vi "Obtain Events.vi"(8 "Error In":errorcluster, 11 "SPD.Stand Ctrl in":T1 {"spdDeviceSession"."hidSPD.Controller"."HV_bias" format="%#_6p, V"; "spdDeviceSession"."hidSPD.Controller"."TSet" format="%#_6p, DegC"}) -> (0 "Error Out":errorcluster, 2 "Event Registration Refnum":refnum<event-registration>, 3 "SPD.Stand Ctrl out":T1 {"spdDeviceSession"."hidSPD.Controller"."HV_bias" format="%#_6p, V"; "spdDeviceSession"."hidSPD.Controller"."TSet" format="%#_6p, DegC"})   [LabVIEW 2018]
uses:
  typedefs/SPD.Stand Ctrl.ctl
  Instruments/SPD HID Interface/hidSPDLibForLabView/LibVIs/hidSPD Controls/hidSPD Device Session.ctl
  Instruments/SPD HID Interface/hidSPDLibForLabView/LibVIs/hidSPD Controls/hidSPD Controller.ctl
  Instruments/KC705 DevBoard/typedefs/DevB.Session.ctl
  Instruments/KeySight 53230A/typedefs/FreqC.Session.ctl
  Instruments/KeySight 8164B/KeySight 8164B LAN InstrLib/typedefs/KeySight 8164B control.ctl
  Instruments/LeCroy SDA830/typedefs/LeCroy.Session.ctl
  typedefs/SPD.Events.ctl
  <vilib>/Utility/config.llb/Config Data RefNum.ctl
  typedefs/SPD.Meas Result.ctl
  Instruments/SPD HID Interface/hidSPDLibForLabView/hidSPDLibForLabView.lvlib
  Instruments/KeySight 8164B/KeySight 8164B LAN InstrLib.lvlib
  <vilib>/Utility/config.llb/NI_LVConfig.lvlib
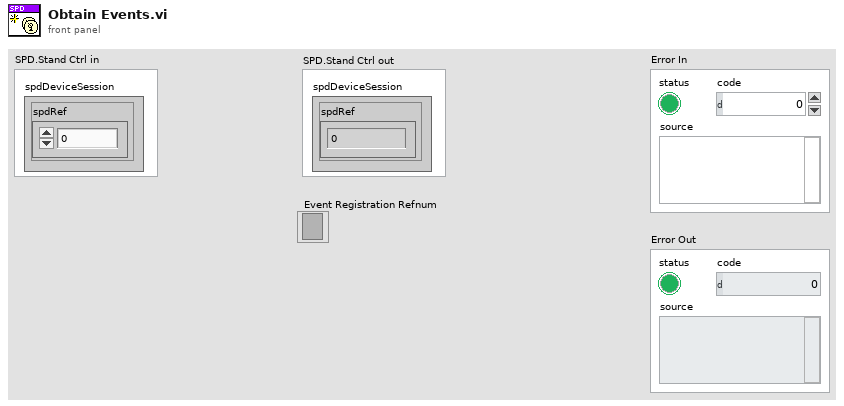
[diagram p1: front panel]
types:
  T1 = typedef "SPD.Stand Ctrl.ctl" = cluster{"spdDeviceSession":T2, "DevBSession":T4, "FreqCSession":T5, "8164BSession":T6, "LeCroySession":T7, "Events":T8, "configFile":T9, "SPD.Result":T10}
  T2 = typedef "hidSPDLibForLabView.lvlib/hidSPD Device Session.ctl" = cluster{"spdRef":u64, "connected":bool, "spdName":string, "hidSPD.Controller":T3}
  T3 = typedef "hidSPDLibForLabView.lvlib/hidSPD Controller.ctl" = cluster{"TSet":sgl, "HV_bias":sgl, "DDS_stb_code":u16}
  T4 = typedef "DevB.Session.ctl" = cluster{"DevBRef":refnum<visa-resource-name>, "connected":bool}
  T5 = typedef "FreqC.Session.ctl" = cluster{"FreqCRef":refnum<visa-resource-name>, "timeout":dbl, "connected":bool}
  T6 = typedef "KeySight 8164B LAN InstrLib.lvlib/KeySight 8164B control.ctl" = cluster{"Connection ID":refnum<k5>, "Connected":bool, "Info":string, "Slots Info":string[]}
  T7 = typedef "LeCroy.Session.ctl" = cluster{"LeCroySession":refnum<visa-resource-name>, "connected":bool}
  T8 = typedef "SPD.Events.ctl" = cluster{"DCRTest":refnum<user-event>, "Stop":refnum<user-event>}
  T9 = typedef "NI_LVConfig.lvlib/Config Data RefNum.ctl" = refnum<k1>
  T10 = typedef "SPD.Meas Result.ctl" = cluster{"HV_Bias":dbl[], "Stb_code":dbl[], "Temprature":dbl[], "Data":dbl[][][][]}
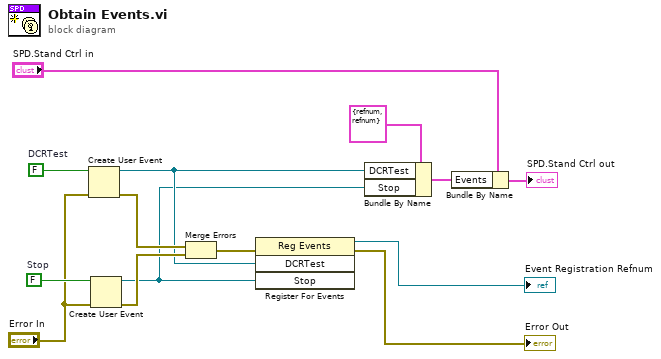
[diagram p0: block diagram]
diagram:
  w6 = FALSE  # Stop
  w14 = FALSE  # DCRTest
  n1 = Create User Event(user event datatype=w14, error in="Error In") -> (user event=w2:refnum<user-event>, error out=w10:errorcluster)
  n2 = Create User Event(user event datatype=w6, error in="Error In") -> (user event=w1:refnum<user-event>, error out=w3:errorcluster)
  n3 = Merge Errors(w10, w3) -> (w4:errorcluster)
  n4 = register-events(error in=w4, w2, w1) -> (reference out=→"Event Registration Refnum":refnum<event-registration>, error out=→"Error Out":errorcluster)  [unwired: 1 in]
  n5 = Bundle By Name(cluster=T8 {"DCRTest"=refnum, "Stop"=refnum} ("Events Cluster"), "DCRTest"=w2, "Stop"=w1) -> (w11:T8)
  n6 = Bundle By Name(cluster="SPD.Stand Ctrl in", "Events"=w11) -> (→"SPD.Stand Ctrl out":T1)
